vi "Math-NaN Mean.vi"(1 "Array":dbl[](array[numeric])) -> (0 "NaN Mean":dbl)   [LabVIEW 2020]
uses:
  <vilib>/Analysis/baseanly.llb/Mean (DBL).vi
  <vilib>/Analysis/NI_AALBase.lvlib
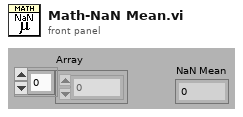
[diagram p1: front panel]
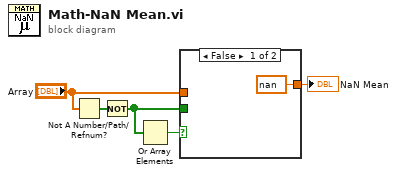
[diagram p0: block diagram]
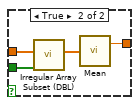
[diagram p2: hidden frame]
diagram:
  n1 = Not A Number/Path/Refnum?(number/path/refnum="Array") -> (NaN/Path/Refnum?=w3:bool[])
  n2 = Not(x=w3) -> (.not. x?=w2:bool[])
  n3 = Or Array Elements(Boolean array=w2) -> (logical OR=w1:bool)
  n4 = case shown="False" w1 {
    tunnel: [nan ("mean") w10] -> w5
    tunnel: "Array" -> [_ w9]
    tunnel: w2 -> [_ w7]
    frame False {
    }
    frame True {
      n5 = call "Irregular Array Subset (DBL).vi"("Mask"=w7, "Array"=w9) -> ("Array Subset"=w8:dbl[])  [unwired: 8 in, 1 out]
      n6 = call-poly <vilib>:"Mean.vi"("X"=w8) -> ("mean"=w10:dbl)  [unwired: 1 out]
    }
  }
  "NaN Mean" <- w5
